vi "DriveGlobal.vi"() -> ()   [LabVIEW 2014]
panel:
  out "Drive speeds":T1
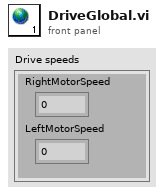
[diagram p1: front panel]
types:
  T1 = cluster{"RightMotorSpeed":dbl, "LeftMotorSpeed":dbl}
diagram:
